vi "CoboltLaser_FaultOperatingGet.vi"(0 "ComPort":refnum<visa-resource-name>, 3 "CheckResponse":bool=TRUE, 7 "error in (no error)":errorcluster) -> (20 "ComPortOut":refnum<visa-resource-name>, 21 "Fault":string, 27 "error out":errorcluster)   [LabVIEW 2019]
doc: "Use this template to build a VI to use as a subVI."
panel:
  out "ResponseOK":bool
  out "Response":string
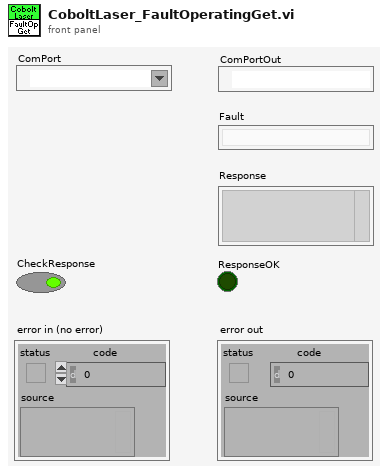
[diagram p1: front panel]
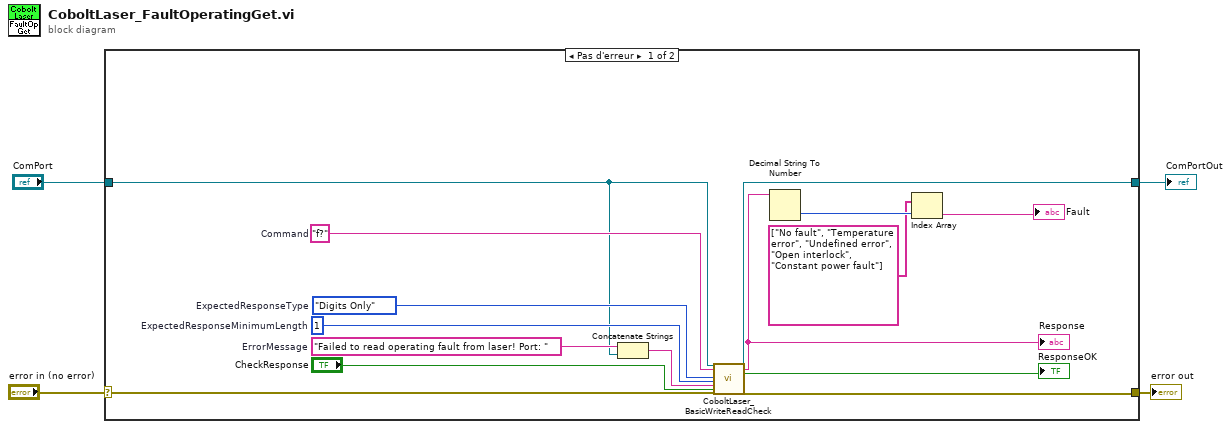
[diagram p0: block diagram]
diagram:
  n1 = case shown="Pas d'erreur" "error in (no error)" {
    selector: "error in (no error)" -> [w19 w21]
    tunnel: [w18 w21] -> w3
    tunnel: "ComPort" -> [w6 w20]
    tunnel: [w5 w20] -> w1
    frame No Error {
      w15 = 1  # ExpectedResponseMinimumLength
      w16 = enum16{"Any", "Digits Only", "Non-Digits Only"}."Digits Only"  # ExpectedResponseType
      w12 = "Failed to read operating fault from laser! Port: "  # ErrorMessage
      w17 = "f?"  # Command
      n2 = Concatenate Strings(w12, w6) -> (w11:string)
      n3 = call <userlib>:"CoboltLaser_BasicWriteReadCheck.vi"("ComPort"=w6, "Command"=w17, "ExpectedResponseType"=w16, "ExpectedResponseMinimumLength"=w15, "ErrorMessage"=w11, "GenerateError"="CheckResponse", "error in (no error)"=w19) -> ("ComPortOut"=w5:refnum<visa-resource-name>, "Response"=w10:string, "ResponseOK"=→"ResponseOK":bool, "error out"=w18:errorcluster)  [unwired: 17 in]
      "Response" <- w10
      n4 = Decimal String To Number(string=w10) -> (number=w9:i32)  [unwired: 2 in, 1 out]
      n5 = Index Array(array=string[] ["No fault", "Temperature error", "Undefined error", "Open interlock", "Constant power fault"], index=w9) -> (element=→"Fault":string)
    }
    frame Error {
    }
  }
  "error out" <- w3
  "ComPortOut" <- w1
